vi "parse_vector3.vi"(4 "error in":errorcluster, 7 "msg in":string) -> (0 "error out":errorcluster, 2 "Vector3":cluster{"x":dbl, "y":dbl, "z":dbl}, 3 "msg out":string)   [LabVIEW 2010]
uses:
  primitives/subs/parse_float64_scalar.vi
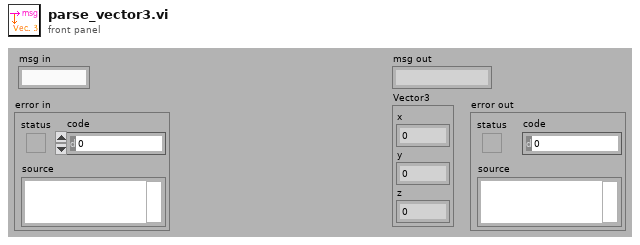
[diagram p1: front panel]
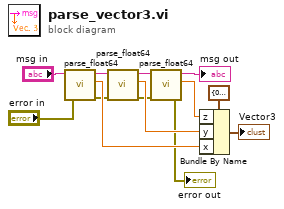
[diagram p0: block diagram]
diagram:
  n1 = call-poly "parse_float64.vi"("error in"="error in", "msg in"="msg in") -> ("error out"=w4:errorcluster, "number"=w8:dbl, "msg out"=w13:string)  [unwired: 3 in]
  n2 = call-poly "parse_float64.vi"("error in"=w4, "msg in"=w13) -> ("error out"=w3:errorcluster, "number"=w9:dbl, "msg out"=w12:string)  [unwired: 3 in]
  n3 = call-poly "parse_float64.vi"("error in"=w3, "msg in"=w12) -> ("error out"=→"error out":errorcluster, "number"=w10:dbl, "msg out"=→"msg out":string)  [unwired: 3 in]
  n4 = Bundle By Name(cluster=cluster{"x":dbl, "y":dbl, "z":dbl} {"x"=0.0, "y"=0.0, "z"=0.0} ("Point32"), "z"=w10, "y"=w9, "x"=w8) -> (→"Vector3":cluster{"x":dbl, "y":dbl, "z":dbl})
